vi "SubVI_GetHumidity.vi"(11 "ErrorIn":errorcluster) -> (1 "fHumidity":sgl, 3 "ErrorOut":errorcluster, 4 "u8Error":u8)   [LabVIEW 2013]
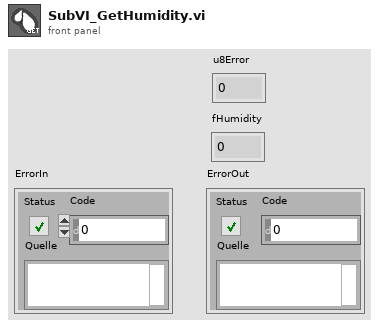
[diagram p1: front panel]
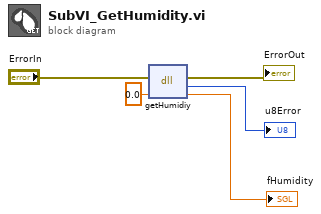
[diagram p0: block diagram]
diagram:
  n1 = dll-call lib="PTH1abs CUsers1000len-bimDesktop&Lieferung_LabView_Interface_11.11.2015Einrichten fÃ¼r - EndkundenDatenTesto_v2013VIlabview_cwrapper_1_0_0.dll" fn="getHumidiy"(error in="ErrorIn", "fHumidity"=sgl 0.0) -> (error out=→"ErrorOut":errorcluster, "u8Error"=→"u8Error":u8, "fHumidity"=→"fHumidity":sgl)  [unwired: 2 in, 1 out]
